vi "Configure Auth.vi"(5 "Optional Providers (Basic)":T3, 6 "Role Hierarchy (None)":T1[](array[typedef]), 7 "User Type":refnum<class "User.lvclass">, 8 "error in":errorcluster, 9 "Auth Handlers (Built-In)":T2, 10 "Entity Manager":refnum<class "Entity Manager.lvclass">, 11 "HTTP Server In":refnum<class "Server.lvclass">) -> (0 "error out":errorcluster, 3 "HTTP Server":refnum<class "Server.lvclass">)   [LabVIEW 2020, in "HTTP-Conditum.lvlib"]
doc: "If this VI is called, <b>Configure Services.vi</b> does not need to be called. This VI registers the provided authentication mechanisms or utilizes HTTP Server built-in defaults and wraps the entity manager instance in a service to be accesible within http handlers.\n\nCall this VI when you want Conditum to manage user entities used with authentication. If conditum entity-based users are not needed then <b>Configure Services.vi</b> should be called instead to allow entity manager access within http requests.\n\nBefore calling this VI, all used entities should be registered with the entity manager instance for best performance."
uses:
  HTTP-Conditum.lvlib
  <vilib>/IlluminatedG/IG HTTP Server/HTTP Server/Server/Server.lvclass
  User Provider/User Provider.lvclass
  <vilib>/IlluminatedG/IG HTTP Server/HTTP Server/Password Encoder/Password Encoder.lvclass
  <vilib>/IlluminatedG/IG HTTP Server/HTTP Server/Authentication Provider/Authentication Provider.lvclass
  <vilib>/IlluminatedG/IG HTTP Server/HTTP Server/Optional Providers.ctl
  <vilib>/IlluminatedG/IG HTTP Server/HTTP Server/HTTP Server.lvlib
  User/User.lvclass
  <vilib>/IlluminatedG/IG Conditum/Conditum/Entity Manager/Entity Manager.lvclass
  <vilib>/IlluminatedG/IG HTTP Server/HTTP Server/Request Handler/Request Handler.lvclass
  <vilib>/IlluminatedG/IG HTTP Server/HTTP Server/Response Handler/Response Handler.lvclass
  <vilib>/IlluminatedG/IG HTTP Server/HTTP Server/Exception Handler/Exception Handler.lvclass
  <vilib>/IlluminatedG/IG HTTP Server/HTTP Server/Auth Handlers.ctl
  <vilib>/IlluminatedG/IG HTTP Server/HTTP Server/Role Inheritance.ctl
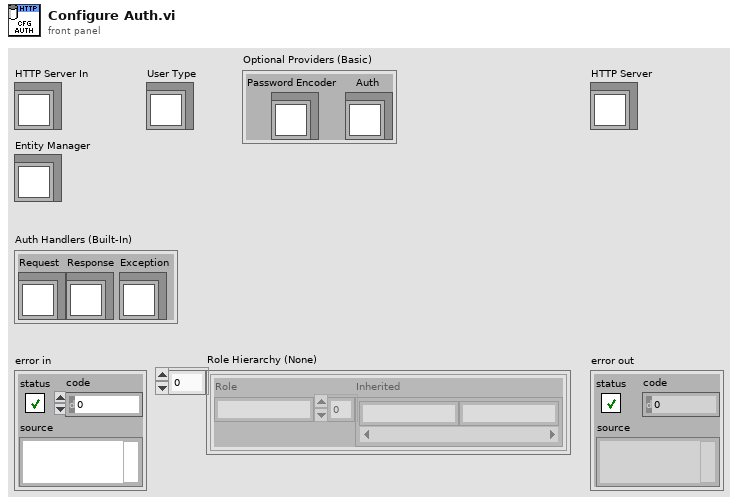
[diagram p1: front panel]
types:
  T1 = typedef "HTTP Server.lvlib/Role Inheritance.ctl" = cluster{"Role":string, "Inherited":string[]}
  T2 = typedef "HTTP Server.lvlib/Auth Handlers.ctl" = cluster{"Request":refnum<class "Request Handler.lvclass">, "Response":refnum<class "Response Handler.lvclass">, "Exception":refnum<class "Exception Handler.lvclass">}
  T3 = typedef "HTTP Server.lvlib/Optional Providers.ctl" = cluster{"Password Encoder":refnum<class "Password Encoder.lvclass">, "Auth":refnum<class "Authentication Provider.lvclass">}
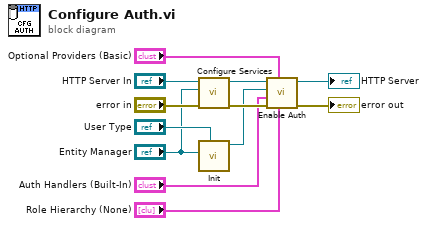
[diagram p0: block diagram]
diagram:
  n1 = call "Configure Services.vi"("error in"="error in", "Entity Manager"="Entity Manager", "HTTP Server In"="HTTP Server In") -> ("error out"=w12:errorcluster, "HTTP Server"=w2:refnum<class "Server.lvclass">)  [unwired: 7 in]
  n2 = call "Init.vi"("User Type"="User Type", "Entity Manager"="Entity Manager") -> ("User Provider out"=w6:refnum<class "User Provider.lvclass">)  [unwired: 9 in]
  n3 = call <vilib>:"Enable Auth.vi"("Role Hierarchy (None)"="Role Hierarchy (None)", "Optional Providers (Basic)"="Optional Providers (Basic)", "error in (no error)"=w12, "Auth Handlers (Built-In)"="Auth Handlers (Built-In)", "User Provider"=w6, "Server in"=w2) -> ("error out"=→"error out":errorcluster, "Server out"=→"HTTP Server":refnum<class "Server.lvclass">)  [unwired: 4 in]
